vi "PreLoop.vi"(6 "Error":errorcluster, 7 "Actor":refnum<class "Actor.lvclass">) -> (5 "Actor":refnum<class "Actor.lvclass">)   [LabVIEW 2020, in "jettl.lvlib" / "Base.lvlib" / "Actor.lvclass"]
uses:
  Actor.lvclass
  Actor.lvclass/Actor.ctl
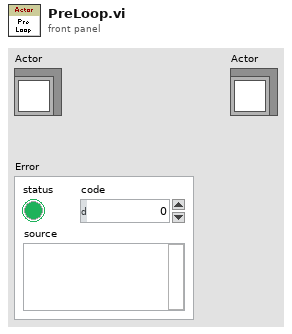
[diagram p1: front panel]
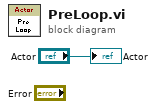
[diagram p0: block diagram]
diagram:
  "Actor" <- "Actor"
